vi "process.vi"(8 "error in (no error)":errorcluster, 10 "array in":u16[](array[numeric]), 11 "cluster in":T1={"reception"={"square length"=3, "offset"=0, "# squares out"=0, "left over"=[], "raps points length"=1}, "fft"={"reference"=[]}}) -> (0 "error out":errorcluster, 2 "manual offset":i16[](array[numeric]), 3 "cluster out":T1={"reception"={"square length"=3, "offset"=0, "# squares out"=0, "left over"=[], "raps points length"=1}, "fft"={"reference"=[]}}, 5 "subarray":dbl[][](array[numeric]))   [LabVIEW 2010]
uses:
  motion_correction_cluster.ctl
  <vilib>/Analysis/2dsp.llb/2D Real FFT.vi
  <vilib>/Analysis/2dsp.llb/2D Inverse Real FFT.vi
  <vilib>/Analysis/NI_AALPro.lvlib
panel:
  out "double precision float":dbl[][][](array[numeric])
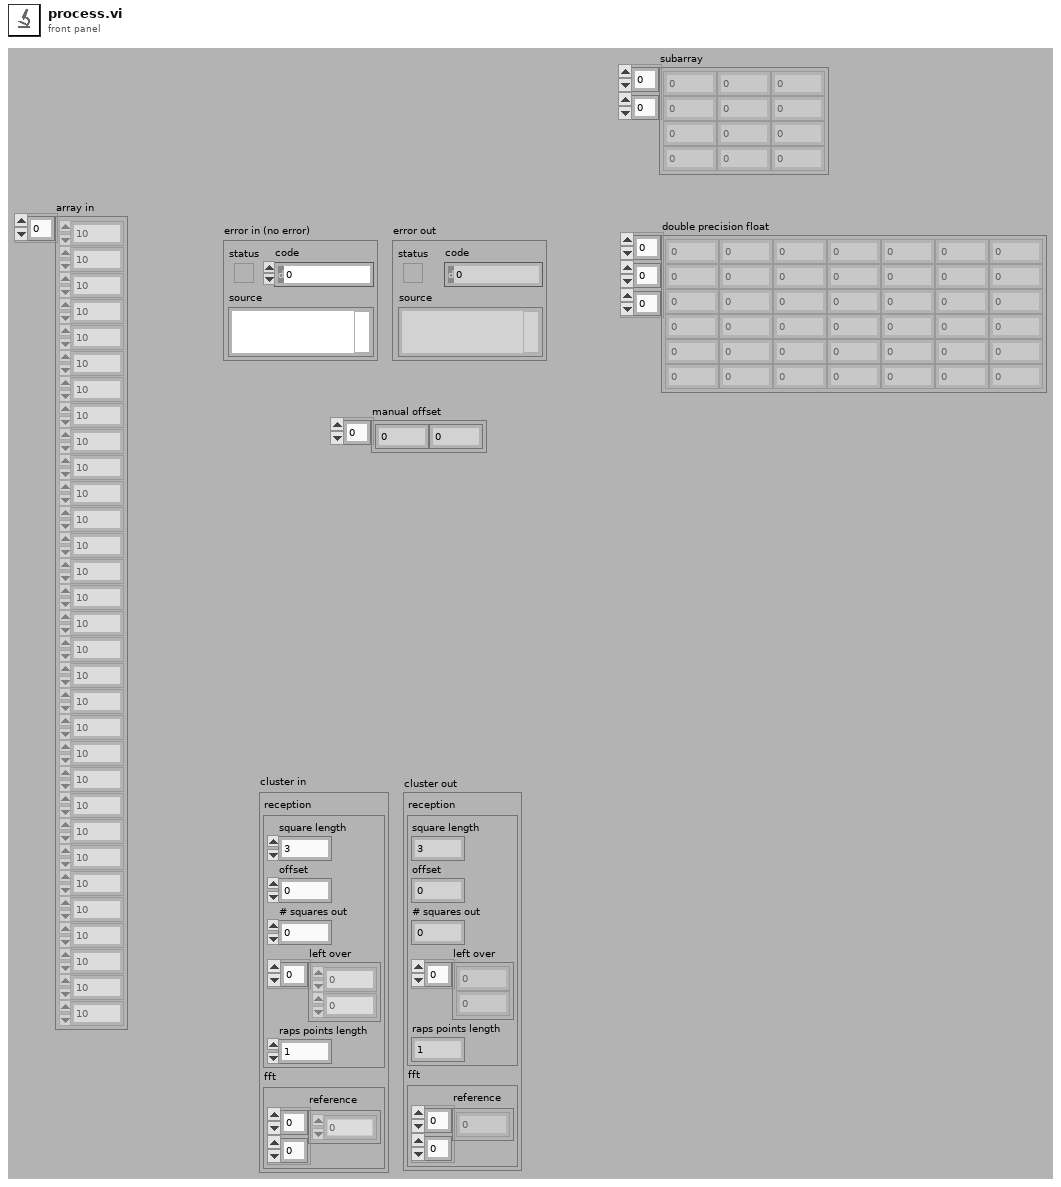
[diagram p1: front panel]
types:
  T1 = typedef "motion_correction_cluster.ctl" = cluster{"reception":cluster{"square length":i32, "offset":i32, "# squares out":i32, "left over":u16[], "raps points length":i32}, "fft":cluster{"reference":dbl[][]}}
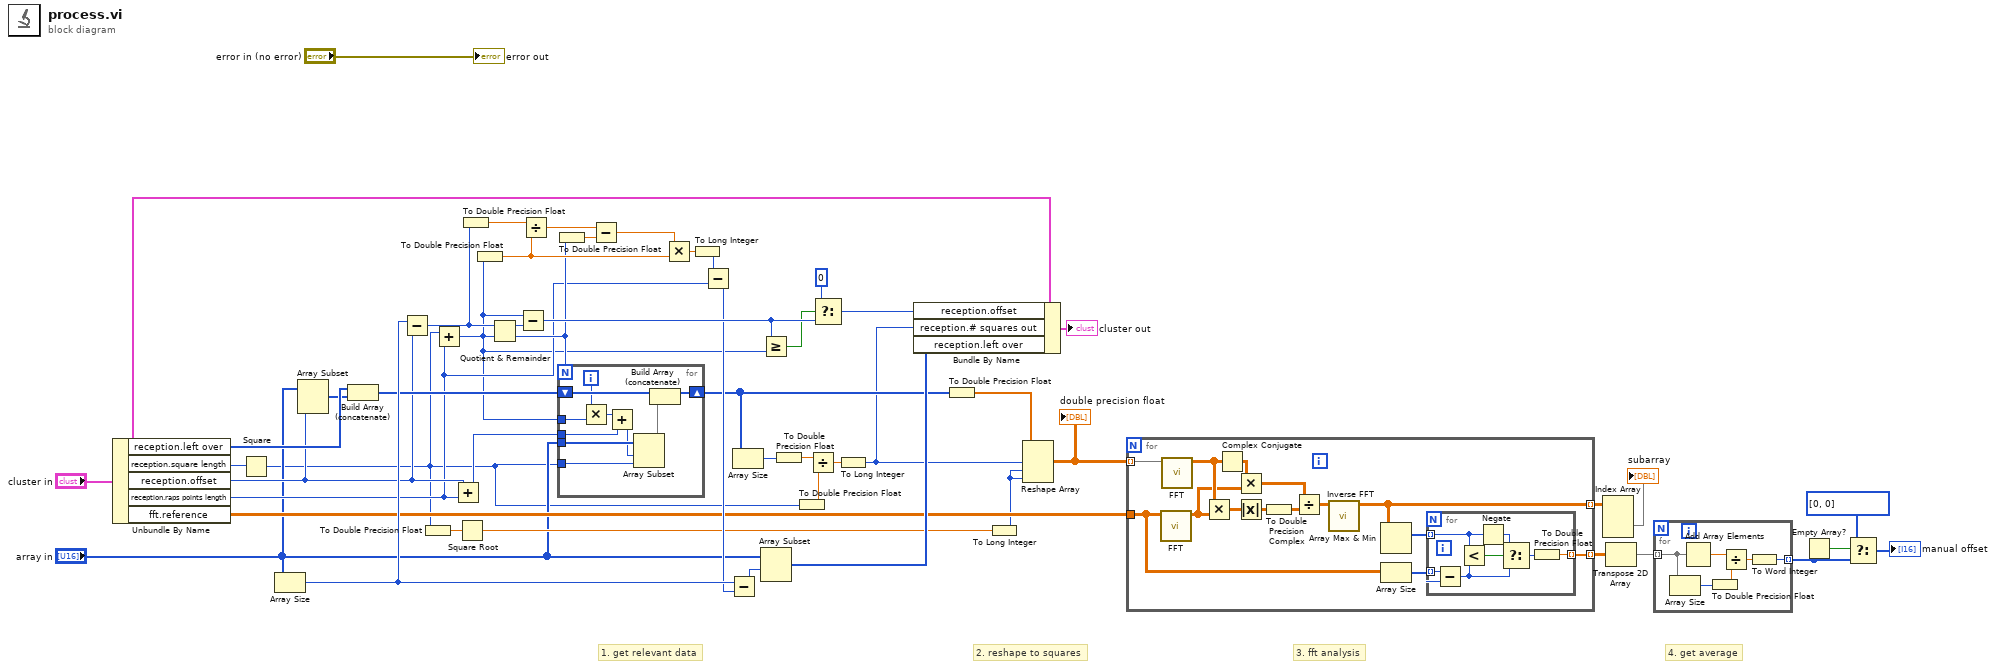
[diagram p0: block diagram]
diagram:
  # "4. get average"
  # "3. fft analysis"
  # "2. reshape to squares"
  # "1. get relevant data"
  n1 = Unbundle By Name("cluster in") -> ("reception.left over"=w48:u16[], "reception.square length"=w18:i32, "reception.offset"=w19:i32, "reception.raps points length"=w15:i32, "fft.reference"=w23:dbl[][])
  n2 = Square(x=w18) -> (x^2=w5:i32)
  n3 = Array Size(array="array in") -> (size(s)=w49:i32)
  n4 = Array Subset(array="array in", length=w19) -> (w34:u16[])  [unwired: 1 in]
  n5 = Build Array (concatenate)(w48, w34) -> (w35:u16[])
  n6 = Subtract(x=w49, y=w19) -> (x-y=w27:i32)
  n7 = To Double Precision Float(number=w5) -> (double precision float=w22:dbl)
  n8 = Add(x=w5, y=w15) -> (x+y=w14:i32)
  n9 = Add(x=w19, y=w15) -> (x+y=w26:i32)
  n10 = Square Root(x=w22) -> (sqrt(x)=w21:dbl)
  n11 = To Double Precision Float(number=w27) -> (double precision float=w36:dbl)
  n12 = To Double Precision Float(number=w14) -> (double precision float=w38:dbl)
  n13 = Quotient & Remainder(x=w27, y=w14) -> (x-y*floor(x/y)=w40:i32, floor(x/y)=w29:i32)
  n14 = Subtract(x=w14, y=w40) -> (x-y=w46:i32)
  n15 = Divide(x=w36, y=w38) -> (x/y=w28:dbl)
  n16 = To Double Precision Float(number=w29) -> (double precision float=w39:dbl)
  n17 = for {
    N: w29 -> [_]
    tunnel: "array in" -> [w61]
    tunnel: w26 -> [w53]
    tunnel: w5 -> [w60]
    shift-right: [w58] -> w20
    shift-left: w35 -> [w57]
    tunnel: w14 -> [w55]
    i -> [w56]
    n18 = Multiply(x=w56, y=w55) -> (x*y=w54:i32)
    n19 = Add(x=w54, y=w53) -> (x+y=w52:i32)
    n20 = Array Subset(array=w61, index=w52, length=w60) -> (w59:u16[])
    n21 = Build Array (concatenate)(w57, w59) -> (w58:u16[])
  }
  n22 = Subtract(x=w28, y=w39) -> (x-y=w30:dbl)
  n23 = Multiply(x=w30, y=w38) -> (x*y=w31:dbl)
  n24 = To Long Integer(number=w31) -> (32bit integer=w37:i32)
  n25 = Subtract(x=w37, y=w15) -> (x-y=w32:i32)
  n26 = Subtract(x=w49, y=w32) -> (x-y=w33:i32)
  n27 = Array Size(array=w20) -> (size(s)=w41:i32)
  n28 = Greater Or Equal?(x=w46, y=w14) -> (x >= y?=w45:bool)
  n29 = Array Subset(array="array in", index=w33) -> (w51:u16[])  [unwired: 1 in]
  n30 = To Double Precision Float(number=w41) -> (double precision float=w43:dbl)
  n31 = To Double Precision Float(number=w5) -> (double precision float=w44:dbl)
  n32 = Divide(x=w43, y=w44) -> (x/y=w42:dbl)
  n33 = Select(t=0, s=w45, f=w46) -> (s? t:f=w50:i32)
  n34 = To Long Integer(number=w42) -> (32bit integer=w17:i32)
  n35 = Bundle By Name(cluster="cluster in", "reception.offset"=w50, "reception.# squares out"=w17, "reception.left over"=w51) -> (→"cluster out":T1)
  n36 = To Double Precision Float(number=w20) -> (double precision float=w10:dbl[])
  n37 = To Long Integer(number=w21) -> (32bit integer=w16:i32)
  n38 = Reshape Array(w10, w17, w16, w16) -> (w9:dbl[][][])
  "double precision float" <- w9
  n39 = for {
    tunnel: w9 -> [w69] mode=indexing
    tunnel: w23 -> [w66]
    tunnel: [w65] -> w11 mode=indexing
    tunnel: [w62] -> w4 mode=indexing
    n40 = call-poly <vilib>:"FFT.vi"("X"=w66) -> ("FFT {X}"=w73:cdb[][])  [unwired: 9 in, 1 out]
    n41 = call-poly <vilib>:"FFT.vi"("X"=w69) -> ("FFT {X}"=w74:cdb[][])  [unwired: 9 in, 1 out]
    n42 = Multiply(x=w74, y=w73) -> (x*y=w70:cdb[][])
    n43 = Complex Conjugate(1:w74) -> (0:w75:cdb[][])
    n44 = Multiply(x=w75, y=w73) -> (x*y=w71:cdb[][])
    n45 = Absolute Value(x=w70) -> (abs(x)=w64:dbl[][])
    n46 = To Double Precision Complex(1:w64) -> (0:w63:cdb[][])
    n47 = Divide(x=w71, y=w63) -> (x/y=w72:cdb[][])
    n48 = call-poly <vilib>:"Inverse FFT.vi"("FFT {X}"=w72) -> ("X"=w62:dbl[][])  [unwired: 9 in, 1 out]
    n49 = Array Max & Min(array=w62) -> (max index (indices)=w68:i32[])  [unwired: 3 out]
    n50 = Array Size(array=w66) -> (size(s)=w67:i32[])
    n51 = for {
      tunnel: w68 -> [w82] mode=indexing
      tunnel: w67 -> [w81] mode=indexing
      tunnel: [w76] -> w65 mode=indexing
      n52 = Subtract(x=w81, y=w82) -> (x-y=w79:i32)
      n53 = Less?(x=w82, y=w79) -> (x < y?=w77:bool)
      n54 = Negate(x=w82) -> (-x=w78:i32)
      n55 = Select(t=w78, s=w77, f=w79) -> (s? t:f=w80:i32)
      n56 = To Double Precision Float(number=w80) -> (double precision float=w76:dbl)
    }
  }
  n57 = Index Array(array=w4) -> (element=→"subarray":dbl[][])  [unwired: 3 in]
  n58 = Transpose 2D Array(2D array=w11) -> (transposed array=w13:dbl[][])
  n59 = for {
    tunnel: w13 -> [w87] mode=indexing
    tunnel: [w83] -> w6 mode=indexing
    n60 = Array Size(array=w87) -> (size(s)=w86:i32)
    n61 = Add Array Elements(numeric array=w87) -> (sum=w88:dbl)
    n62 = To Double Precision Float(number=w86) -> (double precision float=w85:dbl)
    n63 = Divide(x=w88, y=w85) -> (x/y=w84:dbl)
    n64 = To Word Integer(number=w84) -> (16bit integer=w83:i16)
  }
  n65 = Empty Array?(array=w6) -> (empty?=w7:bool)
  n66 = Select(t=i16[] [0, 0] ("manual offset"), s=w7, f=w6) -> (s? t:f=→"manual offset":i16[])
  "error out" <- "error in (no error)"
